vi "provide_OME_data.vi"(6 "image ID":string, 8 "error in (no error)":errorcluster, 9 "structuredAttribute string in":string, 10 "OME element in":refnum<class "XMLElement.lvclass">, 11 "ScanModeDL090923Scaffold in":refnum<class "ImagingModeDL090923Scaffold.lvclass">) -> (0 "error out":errorcluster, 1 "structuredAttribute string out":string, 2 "OME element out":refnum<class "XMLElement.lvclass">, 3 "ScanModeDL090923Scaffold out":refnum<class "ImagingModeDL090923Scaffold.lvclass">)   [LabVIEW 2010, in "ImagingModeDL090923Scaffold.lvclass"]
uses:
  ImagingModeDL090923Scaffold.lvclass
  common/classes/XMLElement/XMLElement/XMLElement.lvclass
  GenericImagingMode/GenericImagingMode/GenericImagingMode.lvclass
  common/classes/ErrorController/ErrorController/class_data.vi
  Instrument/GenericInstrument/GenericInstrument/GenericInstrument.lvclass
  ScanHead/GenericScanHead/GenericScanHead/GenericScanHead.lvclass
  DAQ/GenericDAQ/GenericDAQ/GenericDAQ.lvclass
  ImageAssembler/GenericImageAssembler/GenericImageAssembler/GenericImageAssembler.lvclass
  Display/GenericDisplay/GenericDisplay/GenericDisplay.lvclass
  Analyser/GenericAnalyser/GenericAnalyser/GenericAnalyser.lvclass
  Stimulator/GenericStimulator/GenericStimulator/GenericStimulator.lvclass
  common/classes/ErrorController/ErrorController/ErrorController.lvclass
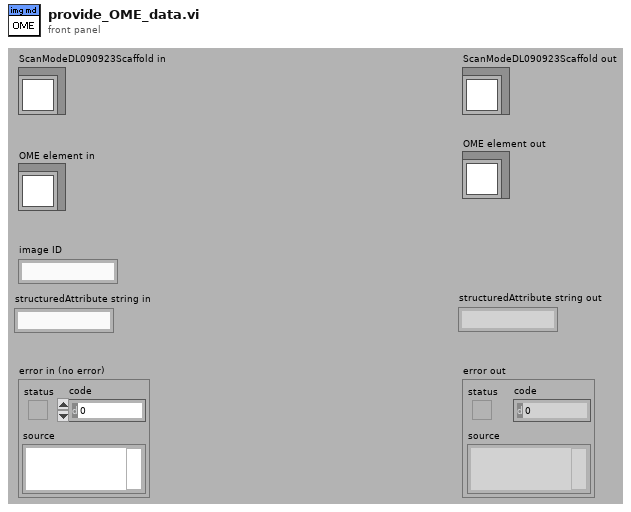
[diagram p1: front panel]
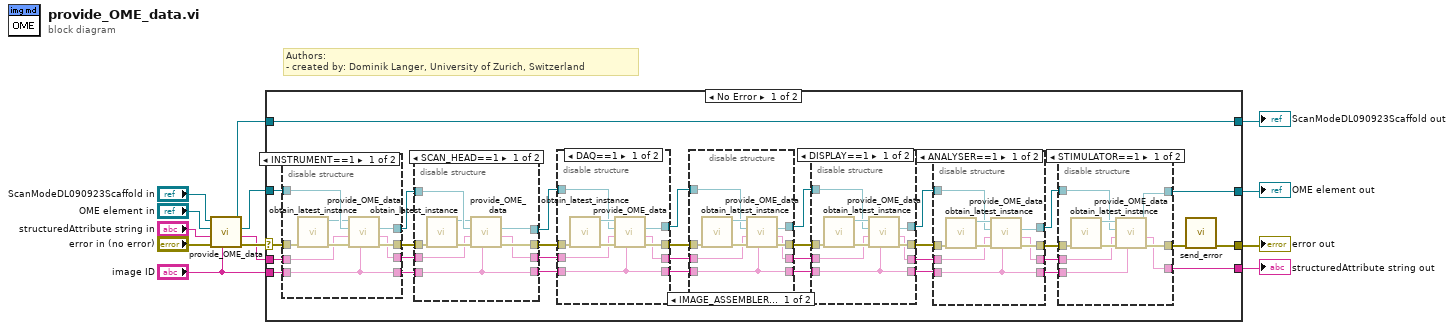
[diagram p0: block diagram]
diagram:
  # "Authors: \n- created by: Dominik Langer, University of Zurich, Switzerland"
  n1 = call-parent "provide_OME_data.vi"("image ID"="image ID", "error in (no error)"="error in (no error)", "structuredAttribute string in"="structuredAttribute string in", "OME element in"="OME element in", "GenericPlugin in"="ScanModeDL090923Scaffold in") -> ("error out"=w10:errorcluster, "structuredAttribute string out"=w2:string, "OME element out"=w8:refnum<class "XMLElement.lvclass">, "GenericPlugin out"=w9:refnum<class "ImagingModeDL090923Scaffold.lvclass">)  [unwired: 3 in]
  n2 = case shown="No Error" w10 {
    selector: w10 -> [w46 w139]
    tunnel: w9 -> [w25 w140]
    tunnel: w8 -> [w45 w138]
    tunnel: "image ID" -> [w44 _]
    tunnel: [w25 w140] -> w7
    tunnel: [w23 w139] -> w6
    tunnel: [w24 w138] -> w5
    tunnel: w2 -> [w21 w137]
    tunnel: [w14 w137] -> w1
    frame No Error {
      n3 = disable-structure shown="INSTRUMENT==1" {
        disable-tunnel: w46 -> [w132 w136]
        disable-tunnel: w45 -> [w130 w134]
        disable-tunnel: w44 -> [w126 w135]
        disable-tunnel: [w128 w136] -> w43
        disable-tunnel: [w126 w135] -> w42
        disable-tunnel: [w127 w134] -> w29
        disable-tunnel: w21 -> [w125 w133]
        disable-tunnel: [w124 w133] -> w20
        frame condition #0 {
          n4 = call "obtain_latest_instance.vi"("error in (no error)"=w132) -> ("error out"=w131:errorcluster, "microscope"=w129:refnum<class "GenericInstrument.lvclass">)  [unwired: 9 in]
          n5 = call-dynamic "provide_OME_data.vi"("image ID"=w126, "error in (no error)"=w131, "structuredAttribute string in"=w125, "OME element in"=w130, "GenericPlugin in"=w129) -> ("error out"=w128:errorcluster, "structuredAttribute string out"=w124:string, "OME element out"=w127:refnum<class "XMLElement.lvclass">)  [unwired: 3 in, 1 out]
        }
        frame condition #1 (active) {
        }
      }
      n6 = disable-structure shown="SCAN_HEAD==1" {
        disable-tunnel: w43 -> [w119 w122]
        disable-tunnel: w42 -> [w113 w121]
        disable-tunnel: w29 -> [w118 w123]
        disable-tunnel: [w115 w122] -> w41
        disable-tunnel: [w114 w123] -> w40
        disable-tunnel: [w113 w121] -> w39
        disable-tunnel: w20 -> [w112 w120]
        disable-tunnel: [w111 w120] -> w19
        frame condition #0 {
          n7 = call "obtain_latest_instance.vi"("error in (no error)"=w119) -> ("error out"=w117:errorcluster, "GenericScanHead out"=w116:refnum<class "GenericScanHead.lvclass">)  [unwired: 9 in]
          n8 = call-dynamic "provide_OME_data.vi"("image ID"=w113, "error in (no error)"=w117, "structuredAttribute string in"=w112, "OME element in"=w118, "GenericScanHead in"=w116) -> ("error out"=w115:errorcluster, "structuredAttribute string out"=w111:string, "OME element out"=w114:refnum<class "XMLElement.lvclass">)  [unwired: 3 in, 1 out]
        }
        frame condition #1 (active) {
        }
      }
      n9 = disable-structure shown="DAQ==1" {
        disable-tunnel: w41 -> [w104 w110]
        disable-tunnel: w40 -> [w103 w109]
        disable-tunnel: w39 -> [w100 w108]
        disable-tunnel: [w102 w110] -> w37
        disable-tunnel: [w101 w109] -> w36
        disable-tunnel: [w100 w108] -> w38
        disable-tunnel: w19 -> [w99 w107]
        disable-tunnel: [w98 w107] -> w18
        frame condition #0 {
          n10 = call "obtain_latest_instance.vi"("error in (no error)"=w104) -> ("error out"=w106:errorcluster, "GenericDAQ out"=w105:refnum<class "GenericDAQ.lvclass">)  [unwired: 9 in]
          n11 = call-dynamic "provide_OME_data.vi"("image ID"=w100, "error in (no error)"=w106, "structuredAttribute string in"=w99, "OME element in"=w103, "GenericPlugin in"=w105) -> ("error out"=w102:errorcluster, "structuredAttribute string out"=w98:string, "OME element out"=w101:refnum<class "XMLElement.lvclass">)  [unwired: 3 in, 1 out]
        }
        frame condition #1 (active) {
        }
      }
      n12 = disable-structure shown="IMAGE_ASSEMBLER==1" {
        disable-tunnel: w37 -> [w91 w97]
        disable-tunnel: w36 -> [w90 w96]
        disable-tunnel: w38 -> [w87 w95]
        disable-tunnel: [w89 w97] -> w34
        disable-tunnel: [w88 w96] -> w33
        disable-tunnel: [w87 w95] -> w35
        disable-tunnel: w18 -> [w86 w94]
        disable-tunnel: [w85 w94] -> w17
        frame condition #0 {
          n13 = call "obtain_latest_instance.vi"("error in (no error)"=w91) -> ("error out"=w93:errorcluster, "GenericImageAssembler out"=w92:refnum<class "GenericImageAssembler.lvclass">)  [unwired: 9 in]
          n14 = call-dynamic "provide_OME_data.vi"("image ID"=w87, "error in (no error)"=w93, "structuredAttribute string in"=w86, "OME element in"=w90, "GenericPlugin in"=w92) -> ("error out"=w89:errorcluster, "structuredAttribute string out"=w85:string, "OME element out"=w88:refnum<class "XMLElement.lvclass">)  [unwired: 3 in, 1 out]
        }
        frame condition #1 (active) {
        }
      }
      n15 = disable-structure shown="DISPLAY==1" {
        disable-tunnel: w34 -> [w78 w84]
        disable-tunnel: w33 -> [w77 w83]
        disable-tunnel: w35 -> [w74 w82]
        disable-tunnel: [w76 w84] -> w32
        disable-tunnel: [w75 w83] -> w30
        disable-tunnel: [w74 w82] -> w31
        disable-tunnel: w17 -> [w73 w81]
        disable-tunnel: [w72 w81] -> w16
        frame condition #0 {
          n16 = call "obtain_latest_instance.vi"("error in (no error)"=w78) -> ("error out"=w80:errorcluster, "GenericDisplay out"=w79:refnum<class "GenericDisplay.lvclass">)  [unwired: 9 in]
          n17 = call-dynamic "provide_OME_data.vi"("image ID"=w74, "error in (no error)"=w80, "structuredAttribute string in"=w73, "OME element in"=w77, "GenericPlugin in"=w79) -> ("error out"=w76:errorcluster, "structuredAttribute string out"=w72:string, "OME element out"=w75:refnum<class "XMLElement.lvclass">)  [unwired: 3 in, 1 out]
        }
        frame condition #1 (active) {
        }
      }
      n18 = disable-structure shown="ANALYSER==1" {
        disable-tunnel: w32 -> [w65 w71]
        disable-tunnel: w30 -> [w64 w70]
        disable-tunnel: w31 -> [w61 w69]
        disable-tunnel: [w63 w71] -> w28
        disable-tunnel: [w62 w70] -> w26
        disable-tunnel: [w61 w69] -> w27
        disable-tunnel: w16 -> [w60 w68]
        disable-tunnel: [w59 w68] -> w15
        frame condition #0 {
          n19 = call "obtain_latest_instance.vi"("error in (no error)"=w65) -> ("error out"=w67:errorcluster, "GeneralAnalyser out"=w66:refnum<class "GenericAnalyser.lvclass">)  [unwired: 9 in]
          n20 = call-dynamic "provide_OME_data.vi"("image ID"=w61, "error in (no error)"=w67, "structuredAttribute string in"=w60, "OME element in"=w64, "GenericPlugin in"=w66) -> ("error out"=w63:errorcluster, "structuredAttribute string out"=w59:string, "OME element out"=w62:refnum<class "XMLElement.lvclass">)  [unwired: 3 in, 1 out]
        }
        frame condition #1 (active) {
        }
      }
      n21 = disable-structure shown="STIMULATOR==1" {
        disable-tunnel: w28 -> [w53 w58]
        disable-tunnel: w26 -> [w52 w57]
        disable-tunnel: w27 -> [w49 _]
        disable-tunnel: [w51 w58] -> w22
        disable-tunnel: [w50 w57] -> w24
        disable-tunnel: w15 -> [w48 w56]
        disable-tunnel: [w47 w56] -> w14
        frame condition #0 {
          n22 = call "obtain_latest_instance.vi"("error in (no error)"=w53) -> ("error out"=w55:errorcluster, "GenericStimulator out"=w54:refnum<class "GenericStimulator.lvclass">)  [unwired: 9 in]
          n23 = call-dynamic "provide_OME_data.vi"("image ID"=w49, "error in (no error)"=w55, "structuredAttribute string in"=w48, "OME element in"=w52, "GenericPlugin in"=w54) -> ("error out"=w51:errorcluster, "structuredAttribute string out"=w47:string, "OME element out"=w50:refnum<class "XMLElement.lvclass">)  [unwired: 3 in, 1 out]
        }
        frame condition #1 (active) {
        }
      }
      n24 = call "send_error.vi"("error in (no error)"=w22) -> ("error out"=w23:errorcluster)  [unwired: 10 in]
    }
    frame Error {
    }
  }
  "error out" <- w6
  "ScanModeDL090923Scaffold out" <- w7
  "OME element out" <- w5
  "structuredAttribute string out" <- w1
